vi "ManipPrespin.vi"(3 "Instruction String":string) -> (0 "Error Out":errorcluster, 1 "Advance Trigger":bool)   [LabVIEW 2020]
doc: "Turns the shooter pre-spin on or off.\n\nParameters: \"on\" or \"off\""
uses:
  SafeParser_String.vi
  autonomousinfo.vi
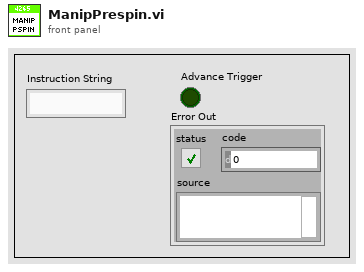
[diagram p1: front panel]
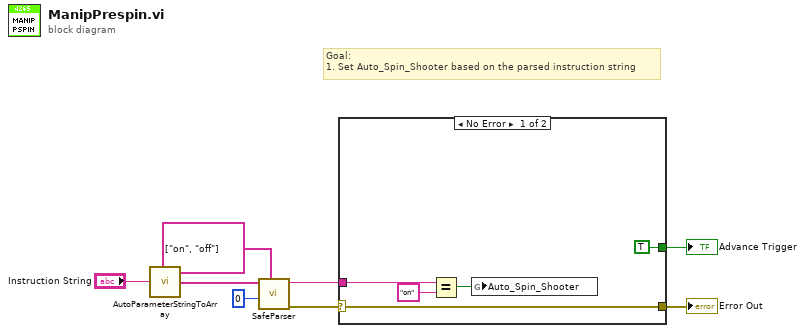
[diagram p0: block diagram]
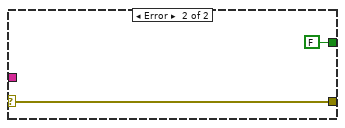
[diagram p2: hidden frame]
diagram:
  # "Goal:\n1. Set Auto_Spin_Shooter based on the parsed instruction string"
  n1 = call "AutoParameterStringToArray.vi"("Parameter String"="Instruction String") -> ("Parsed Parameters"=w5:string[])
  n2 = call-poly "SafeParser.vi"("Allowed Values"=string[] ["on", "off"], "Array Index"=0, "String Array"=w5) -> ("Error Out"=w2:errorcluster, "Typecast Value"=w1:string)  [unwired: 7 in]
  n3 = case shown="No Error" w2 {
    selector: w2 -> [w13 w15]
    tunnel: [TRUE FALSE] -> w8
    tunnel: [w13 w15] -> w7
    tunnel: w1 -> [w11 _]
    frame No Error {
      n4 = Equal?(x=w11, y="on") -> (x = y?=w10:bool)
      n5 = global write "autonomousinfo.vi" "Auto_Spin_Shooter"(w10) -> ()
    }
    frame Error {
    }
  }
  "Advance Trigger" <- w8
  "Error Out" <- w7
